vi "MTM2_getResponse_setLogLevel.vi"(8 "error in (no error)":errorcluster, 11 "ackcmd_Ctl":T1={"private_rcvStamp"=0.0, "cmdSeqNum"=0, "ack"=0, "error"=0, "result"="                                                                                                                                                                                                                                                                ", "host"=0, "identity"="", "origin"=0, "cmdtype"=0, "timeout"=0.0}) -> (0 "error out":errorcluster, 2 "function return":i32, 3 "ackcmd_Ctl out":T1={"private_rcvStamp"=0.0, "cmdSeqNum"=0, "ack"=0, "error"=0, "result"="                                                                                                                                                                                                                                                                ", "host"=0, "identity"="", "origin"=0, "cmdtype"=0, "timeout"=0.0})   [LabVIEW 2018, in "SALLV_MTM2.lvlib"]
doc: "int MTM2_shm_getResponse_setLogLevelLV(MTM2_ackcmdLV *ackcmd_Ctl);"
uses:
  DataTypes/ackcmd.ctl
  SALLV_MTM2.lvlib
  SALLV_MTM2.so
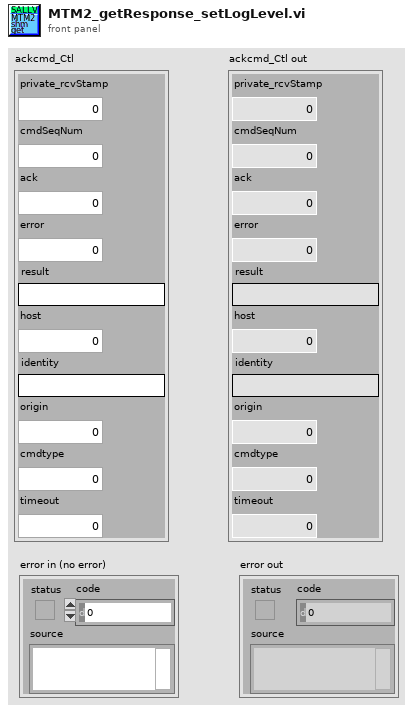
[diagram p1: front panel]
types:
  T1 = typedef "SALLV_MTM2.lvlib/ackcmd.ctl" = cluster{"private_rcvStamp":dbl, "cmdSeqNum":i32, "ack":i32, "error":i32, "result":string, "host":i32, "identity":string, "origin":i32, "cmdtype":i32, "timeout":dbl}
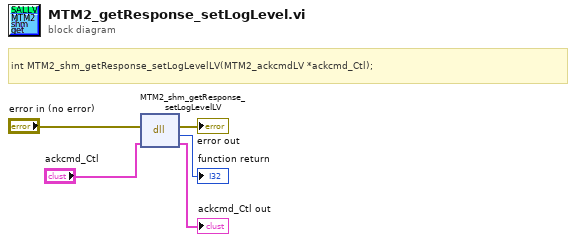
[diagram p0: block diagram]
diagram:
  # "int MTM2_shm_getResponse_setLogLevelLV(MTM2_ackcmdLV *ackcmd_Ctl);"
  n1 = dll-call lib="home/ttsai/Documents/salTestLabViewApi/SALLV_MTM2/SALLV_MTM2.*" fn="MTM2_shm_getResponse_setLogLevelLV"(error in="error in (no error)", "ackcmd_Ctl"="ackcmd_Ctl") -> (error out=→"error out":errorcluster, →"function return":i32, "ackcmd_Ctl"=→"ackcmd_Ctl out":T1)  [unwired: 2 in, 1 out]
